vi "CalculateTempCorrections.vi"(8 "Error In":errorcluster, 10 "Current Tube Temperatures":dbl[](array[numeric]), 11 "Thermistors":i32=2) -> (0 "Error Out":errorcluster, 3 "SSC Out (meters)":dbl[](array[numeric]) format="%_6g")   [LabVIEW 2019, in "Analysis.lvlib"]
doc: "Thermistor locations are hard coded into a constant array with Index 0 at the transducer location. This VI creates weighted temperatures along the length of sounding tube and generates a correction factor in meters to be applied to the final offsets."
uses:
  Analysis/Analysis.lvlib
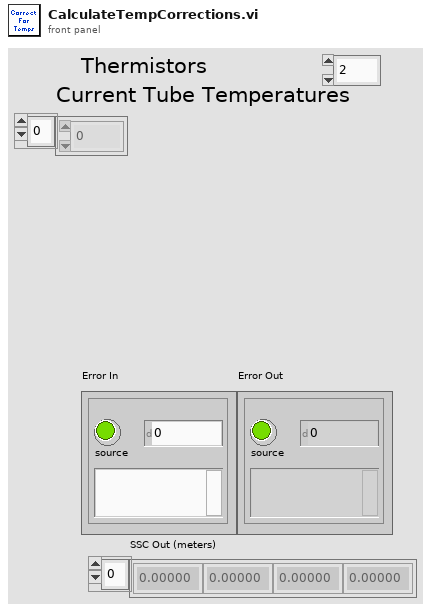
[diagram p1: front panel]
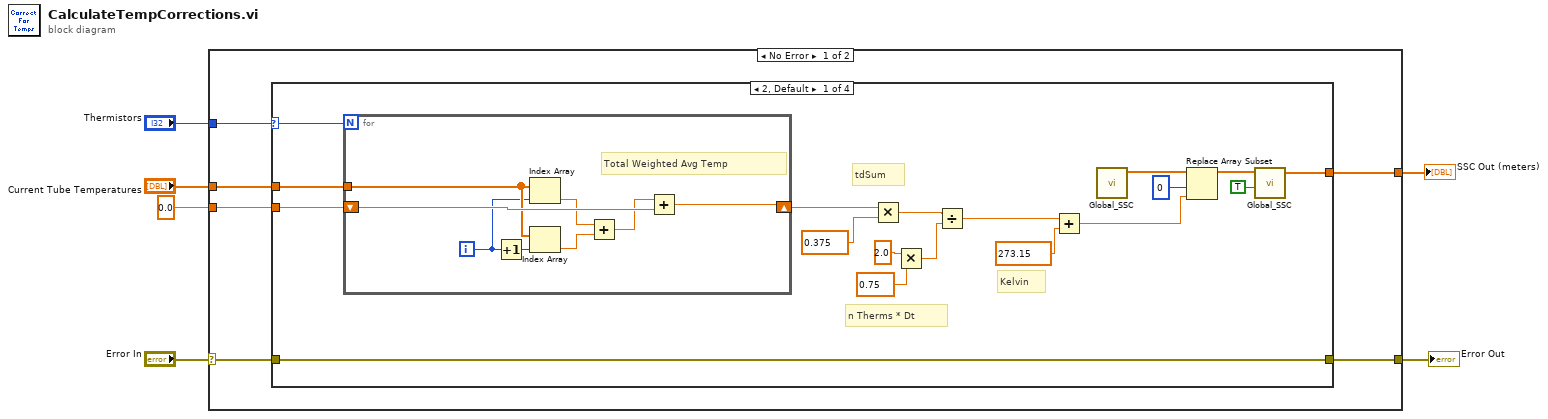
[diagram p0: block diagram]
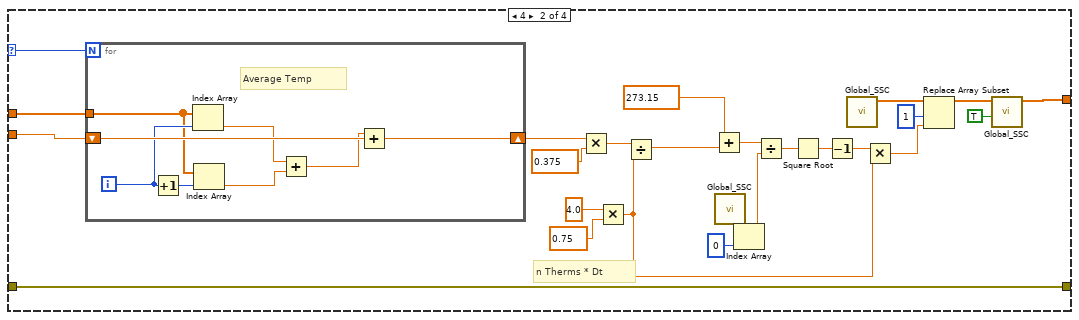
[diagram p2: hidden frame]
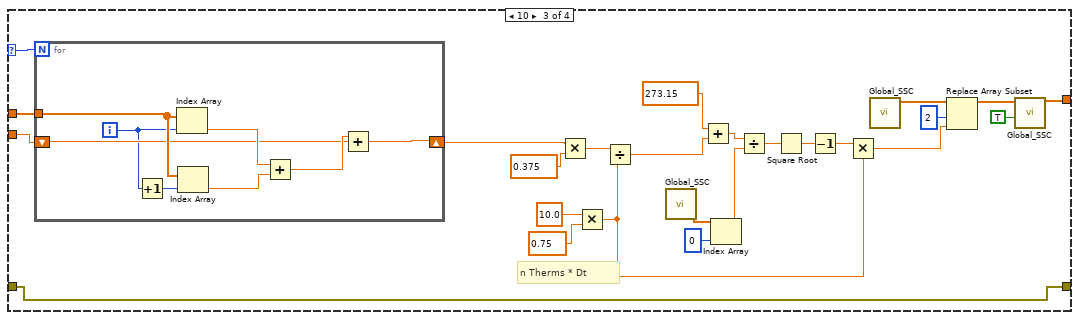
[diagram p3: hidden frame]
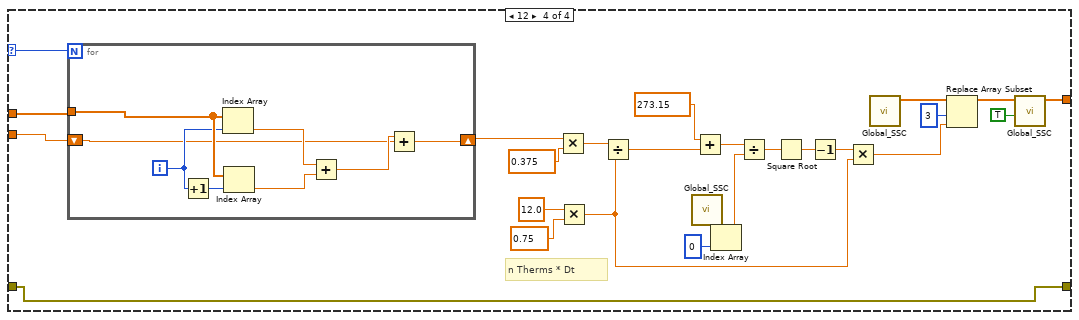
[diagram p4: hidden frame]
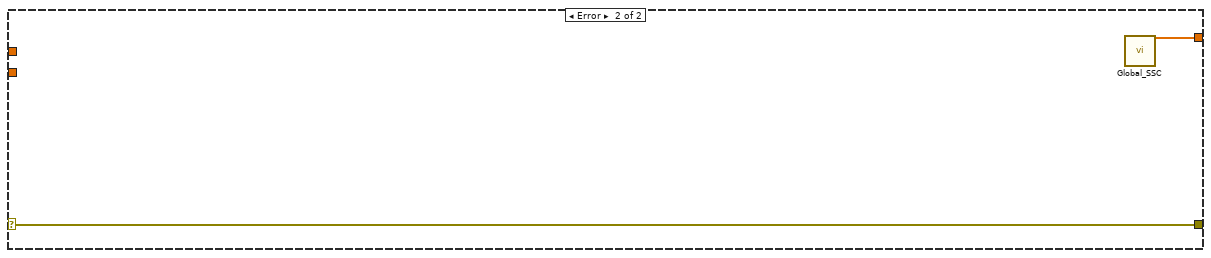
[diagram p5: hidden frame]
diagram:
  n1 = case shown="No Error" "Error In" {
    selector: "Error In" -> [w9 w139]
    tunnel: 0.0 -> [w12 _]
    tunnel: "Current Tube Temperatures" -> [w11 _]
    tunnel: "Thermistors" -> [w10 _]
    tunnel: [w8 w139] -> w3
    tunnel: [w7 w138] -> w2
    frame No Error {
      n2 = case shown="2, Default" w10 {
        selector: w10 -> [w28 w63 w96 w129]
        tunnel: w12 -> [w29 w62 w94 w127]
        tunnel: w11 -> [w30 w61 w95 w128]
        tunnel: w9 -> [w24 w47 w93 w126]
        tunnel: [w24 w47 w93 w126] -> w8
        tunnel: [w22 w52 w79 w112] -> w7
        frame 2, Default {
          # "tdSum"
          # "n Therms * Dt"
          # "Kelvin"
          n3 = for {
            N: w28 -> [_]
            tunnel: w30 -> [w36]
            shift-right: [w37] -> w19
            shift-left: w29 -> [w38]
            i -> [w34]
            # "Total Weighted Avg Temp"
            n4 = Increment(x=w34) -> (x+1=w35:i32)
            n5 = Index Array(array=w36, index=w34) -> (element=w32:dbl)
            n6 = Index Array(array=w36, index=w35) -> (element=w33:dbl)
            n7 = Add(x=w32, y=w33) -> (x+y=w31:dbl)
            n8 = Add(x=w31, y=w38) -> (x+y=w37:dbl)
          }
          n9 = Multiply(x=w19, y=0.375) -> (x*y=w17:dbl)
          n10 = Multiply(x=2.0 ("y"), y=0.75) -> (x*y=w14:dbl)
          n11 = Divide(x=w17, y=w14) -> (x/y=w13:dbl)
          n12 = Add(x=w13, y=273.15) -> (x+y=w20:dbl)
          n13 = call "Global_SSC.vi"() -> ("SSC Out (meters)"=w25:dbl[])  [unwired: 10 in, 1 out]
          n14 = Replace Array Subset(array=w25, new element=w20, index=0) -> (w27:dbl[])
          n15 = call "Global_SSC.vi"("Write?"=TRUE, "SSC In (meters)"=w27) -> ("SSC Out (meters)"=w22:dbl[])  [unwired: 8 in, 1 out]
        }
        frame 4 {
          # "n Therms * Dt"
          n16 = for {
            N: w63 -> [_]
            tunnel: w61 -> [w65]
            shift-right: [w70] -> w45
            shift-left: w62 -> [w71]
            i -> [w68]
            # "Average Temp"
            n17 = Increment(x=w68) -> (x+1=w69:i32)
            n18 = Index Array(array=w65, index=w68) -> (element=w67:dbl)
            n19 = Index Array(array=w65, index=w69) -> (element=w66:dbl)
            n20 = Add(x=w67, y=w66) -> (x+y=w64:dbl)
            n21 = Add(x=w64, y=w71) -> (x+y=w70:dbl)
          }
          n22 = Multiply(x=w45, y=0.375) -> (x*y=w43:dbl)
          n23 = Multiply(x=4.0 ("y"), y=0.75) -> (x*y=w39:dbl)
          n24 = Divide(x=w43, y=w39) -> (x/y=w40:dbl)
          n25 = Add(x=273.15 ("y"), y=w40) -> (x+y=w46:dbl)
          n26 = call "Global_SSC.vi"() -> ("SSC Out (meters)"=w60:dbl[])  [unwired: 10 in, 1 out]
          n27 = Index Array(array=w60, index=0) -> (element=w58:dbl)
          n28 = Divide(x=w46, y=w58) -> (x/y=w50:dbl)
          n29 = Square Root(x=w50) -> (sqrt(x)=w49:dbl)
          n30 = Decrement(x=w49) -> (x-1=w48:dbl)
          n31 = call "Global_SSC.vi"() -> ("SSC Out (meters)"=w56:dbl[])  [unwired: 10 in, 1 out]
          n32 = Multiply(x=w48, y=w39) -> (x*y=w54:dbl)
          n33 = Replace Array Subset(array=w56, new element=w54, index=1) -> (w57:dbl[])
          n34 = call "Global_SSC.vi"("Write?"=TRUE, "SSC In (meters)"=w57) -> ("SSC Out (meters)"=w52:dbl[])  [unwired: 8 in, 1 out]
        }
        frame 10 {
          # "n Therms * Dt"
          n35 = for {
            N: w96 -> [_]
            tunnel: w95 -> [w100]
            shift-right: [w97] -> w75
            shift-left: w94 -> [w99]
            i -> [w98]
            n36 = Increment(x=w98) -> (x+1=w104:i32)
            n37 = Index Array(array=w100, index=w98) -> (element=w103:dbl)
            n38 = Index Array(array=w100, index=w104) -> (element=w102:dbl)
            n39 = Add(x=w103, y=w102) -> (x+y=w101:dbl)
            n40 = Add(x=w101, y=w99) -> (x+y=w97:dbl)
          }
          n41 = Multiply(x=w75, y=0.375) -> (x*y=w78:dbl)
          n42 = Multiply(x=10.0 ("y"), y=0.75) -> (x*y=w73:dbl)
          n43 = Divide(x=w78, y=w73) -> (x/y=w72:dbl)
          n44 = call "Global_SSC.vi"() -> ("SSC Out (meters)"=w92:dbl[])  [unwired: 10 in, 1 out]
          n45 = Add(x=273.15 ("y"), y=w72) -> (x+y=w84:dbl)
          n46 = Index Array(array=w92, index=0) -> (element=w90:dbl)
          n47 = Divide(x=w84, y=w90) -> (x/y=w82:dbl)
          n48 = Square Root(x=w82) -> (sqrt(x)=w81:dbl)
          n49 = Decrement(x=w81) -> (x-1=w80:dbl)
          n50 = Multiply(x=w80, y=w73) -> (x*y=w86:dbl)
          n51 = call "Global_SSC.vi"() -> ("SSC Out (meters)"=w88:dbl[])  [unwired: 10 in, 1 out]
          n52 = Replace Array Subset(array=w88, new element=w86, index=2) -> (w89:dbl[])
          n53 = call "Global_SSC.vi"("Write?"=TRUE, "SSC In (meters)"=w89) -> ("SSC Out (meters)"=w79:dbl[])  [unwired: 8 in, 1 out]
        }
        frame 12 {
          # "n Therms * Dt"
          n54 = for {
            N: w129 -> [_]
            tunnel: w128 -> [w132]
            shift-right: [w133] -> w107
            shift-left: w127 -> [w130]
            i -> [w131]
            n55 = Increment(x=w131) -> (x+1=w137:i32)
            n56 = Index Array(array=w132, index=w131) -> (element=w136:dbl)
            n57 = Index Array(array=w132, index=w137) -> (element=w135:dbl)
            n58 = Add(x=w136, y=w135) -> (x+y=w134:dbl)
            n59 = Add(x=w134, y=w130) -> (x+y=w133:dbl)
          }
          n60 = Multiply(x=w107, y=0.375) -> (x*y=w111:dbl)
          n61 = Multiply(x=12.0 ("y"), y=0.75) -> (x*y=w105:dbl)
          n62 = Divide(x=w111, y=w105) -> (x/y=w106:dbl)
          n63 = call "Global_SSC.vi"() -> ("SSC Out (meters)"=w125:dbl[])  [unwired: 10 in, 1 out]
          n64 = Add(x=273.15 ("y"), y=w106) -> (x+y=w117:dbl)
          n65 = Index Array(array=w125, index=0) -> (element=w123:dbl)
          n66 = Divide(x=w117, y=w123) -> (x/y=w115:dbl)
          n67 = Square Root(x=w115) -> (sqrt(x)=w114:dbl)
          n68 = Decrement(x=w114) -> (x-1=w113:dbl)
          n69 = Multiply(x=w113, y=w105) -> (x*y=w119:dbl)
          n70 = call "Global_SSC.vi"() -> ("SSC Out (meters)"=w121:dbl[])  [unwired: 10 in, 1 out]
          n71 = Replace Array Subset(array=w121, new element=w119, index=3) -> (w122:dbl[])
          n72 = call "Global_SSC.vi"("Write?"=TRUE, "SSC In (meters)"=w122) -> ("SSC Out (meters)"=w112:dbl[])  [unwired: 8 in, 1 out]
        }
      }
    }
    frame Error {
      n73 = call "Global_SSC.vi"() -> ("SSC Out (meters)"=w138:dbl[])  [unwired: 10 in, 1 out]
    }
  }
  "Error Out" <- w3
  "SSC Out (meters)" <- w2
